vi "Constants.vi"() -> ()   [LabVIEW 2014, in "SLSC configuration Shared.lvlib"]
doc: "Use this Global VI to access the GUIDs assigned to the page resources of the Custom Device."
uses:
  SLSC configuration Shared.lvlib
panel:
  in  "Tab Control":T1(tab)=enum."Generic"
  in  "Res Sim Channel":string="c1df0500-e9fe-462d-a67f-7c6056707f28"
  in  "Res Sim Card":string="8c9eb810-a56f-48f6-b7a1-40928e14985f"
  in  "GUID.FIU line":string="419d9b57-9547-4c03-8a6e-b71d44e1efd6"
  in  "GUID.DIO card":string="7fc51c5c-63e7-4d2e-8e21-24b5aba9210e"
  in  "GUID.FIU card":string="8a7a6458-bb89-4ca3-ad7b-82e230caa836"
  in  "SLSC configuration":string="1669feb8-c7a5-4ea6-863a-145b2f30e50b"
  in  "duplicate slot":string="The card slot you selected is already in use. Please select a different slot, or delete the card that has already been added in this slot"
  in  "duplicate name":string="The name you selected is already in use. Please select a different name."
  in  "DIO.Line Config 3":string="DIO Line Config 3"
  in  "DIO.Line Config 2":string="DIO Line Config 2"
  in  "DIO.Line Config 1":string="DIO Line Config 1"
  in  "DIO.Line Config 0":string="DIO Line Config 0"
  in  "DIO.Logic Threshold 3":string="Logic Threshold 3"
  in  "DIO.Logic Threshold 2":string="Logic Threshold 2"
  in  "DIO.Logic Threshold 1":string="Logic Threshold 1"
  in  "DIO.Logic Threshold 0":string="Logic Threshold 0"
  in  "DIO Config":string="DIO Config"
  in  "Generic.Max # of Racks":string="Max # of Racks"
  in  "Generic.SLSC FPGA Settings":string="SLSC FPGA Settings"
  in  "Generic.FIFO Name":string="FIFO Name"
  in  "Generic.Device Settings":string="Device Settings"
  in  "Generic.RIO Dev Address":string="RIO Dev Address"
  in  "Generic.Load Delay":string="Load Delay"
  in  "Generic.Sample Rate":string="Sample Rate"
  in  "Generic.Divide Value":string="Divide Value"
  in  "Generic.Slot #":string="Slot #"
  in  "Generic.Rack #":string="Rack #"
  in  "Generic.Bitfile Path":string="BItfile Path"
  in  "FPGA Name":string="FPGA Name"
  in  "Compiled Info":string="Compiled Info"
  in  "Card Postion":string="Card Position"
  in  "Constants.RT base path":path=path "c:/ni-rt/NIVeriStand/Custom Devices/SLSC"
  in  "Constants.Invalid bitfile":string="Invalid bitfile"
  in  "Constants.FPGA FIFO Name":string="slsc.FIFO Name."
  in  "Constants.FPGA # of racks":string="slsc.# of Racks."
  in  "Constants.# of FIU Channels per Chip":u8=4
  in  "Constants.FIU Chip Addresses":u8[](array[numeric])=[0, 1] format="%02b"
  in  "Constants.DIO Chip Addresses":u8[](array[numeric])=[0, 1, 2, 3] format="%02b"
  in  "Constants.# of Slots":u8=16
  in  "Constants.DIO":string="DIO"
  in  "Constants.# of FIU Channels":u8=8
  in  "Constants.FIU":string="FIU"
  in  "Constants.Sample Rate":string="Sample Rate (S/s)"
  in  "Constants.SPI PHY Settings":string="SPI PHY Settings"
  in  "Constants.DMA FIFO":string="SPI CMD FIFO"
  in  "FIU.Fault #":string="Fault #"
  in  "Channel #":string="Channel number"
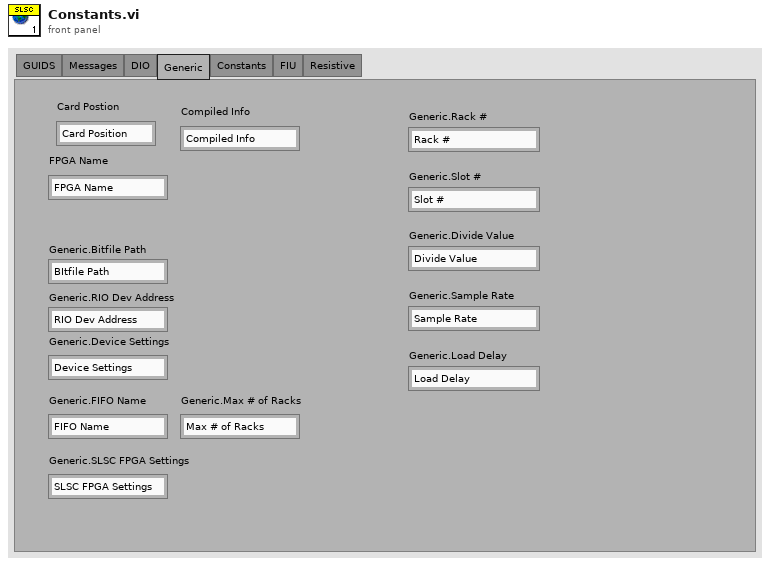
[diagram p1: front panel]
types:
  T1 = enum32{"GUIDS", "Messages", "DIO", "Generic", "Constants", "FIU", "Resistive"}
diagram:
